vi "VSG_SET-GET_CW_1.00.vi"(4 "Set Delay after (ms)":i64 caption="Delay Time (s)", 5 "Skip(T)":bool, 6 "Freq Units":string(combo)="MHz", 7 "Timeout":u32=3000, 8 "error in":errorcluster {"code" format="%.0x"}, 9 "Set Freq (MHz) num":dbl, 10 "Set Freq (MHz)str":string, 11 "Session In":refnum<visa-resource-name>="TCPIP0::10.0.1.20::inst0::INSTR") -> (0 "error out":errorcluster {"code" format="%.0x"}, 1 "Get Freq (str)":string, 2 "Get Freq":dbl, 3 "Session Out":refnum<visa-resource-name>)   [LabVIEW 2018]
doc: "Sets the RF CF in MHz"
panel:
  in  "RO (T)":bool
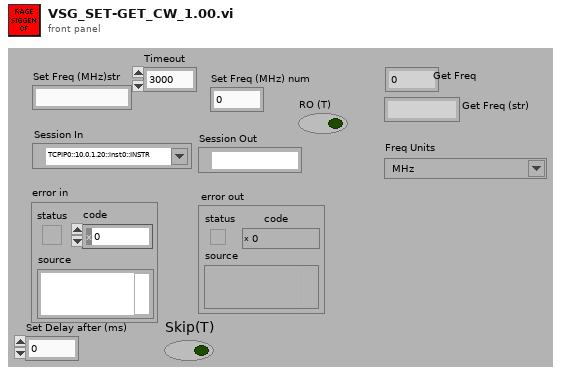
[diagram p1: front panel]
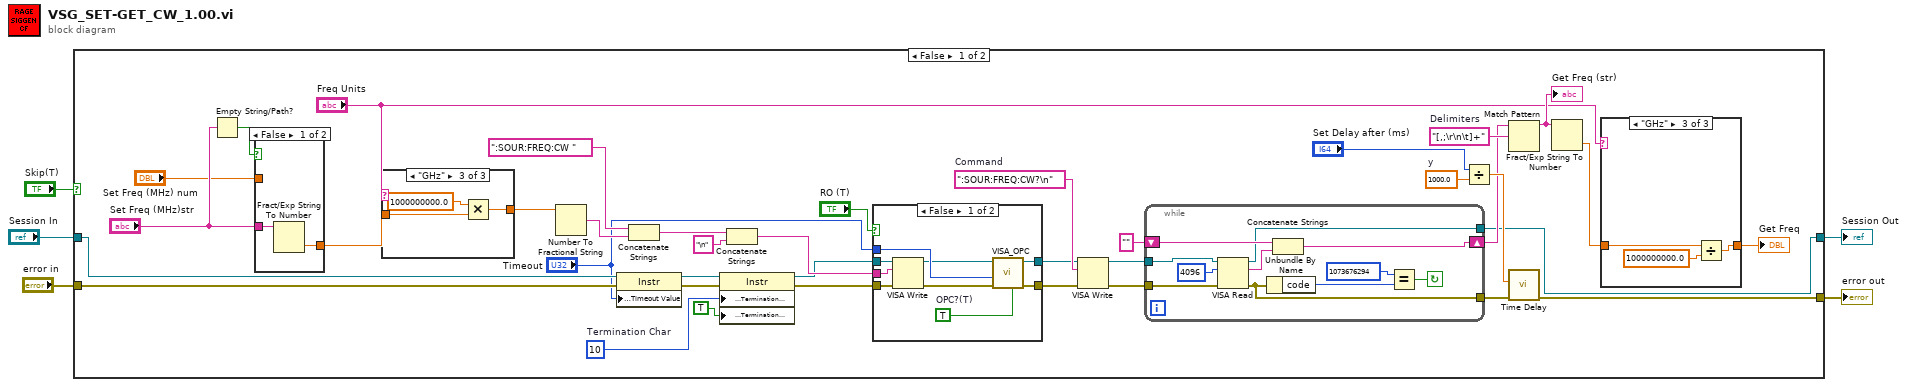
[diagram p0: block diagram]
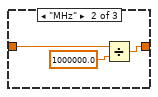
[diagram p4: hidden frame]
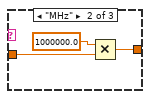
[diagram p6: hidden frame]
diagram:
  n1 = case shown="False" "Skip(T)" {
    tunnel: "error in" -> [w43 w83]
    tunnel: "Session In" -> [w42 w84]
    tunnel: [w6 w84] -> w3
    tunnel: [w16 w83] -> w2
    frame False {
      w13 = 1000.0  # y
      w33 = "[,;\r\n\t]+"  # Delimiters
      w34 = ":SOUR:FREQ:CW?\n"  # Command
      w39 = u8 10  # Termination Char
      n2 = Empty String/Path?(string/path="Set Freq (MHz)str") -> (empty?=w23:bool)
      n3 = case shown="False" w23 {
        tunnel: [w70 w71] -> w28
        tunnel: "Set Freq (MHz)str" -> [w69 _]
        tunnel: "Set Freq (MHz) num" -> [_ w71]
        frame False {
          n4 = Fract/Exp String To Number(string=w69) -> (number=w70:dbl)  [unwired: 3 in, 1 out]
        }
        frame True {
        }
      }
      n5 = case shown="\"GHz\"" "Freq Units" {
        tunnel: w28 -> [w62 w65 w68]
        tunnel: [w62 w63 w66] -> w26
        frame "Hz", Default {
        }
        frame "MHz" {
          n6 = Multiply(x=1000000.0, y=w65) -> (x*y=w63:dbl)
        }
        frame "GHz" {
          n7 = Multiply(x=1000000000.0, y=w68) -> (x*y=w66:dbl)
        }
      }
      n8 = Number To Fractional String(number=w26) -> (F-format string=w27:string)  [unwired: 3 in]
      n9 = property class="Instr"(reference=w42, error in=w43, "General Settings:Timeout Value"="Timeout") -> (reference out=w41:refnum<visa-resource-name>, error out=w40:errorcluster)
      n10 = Concatenate Strings(":SOUR:FREQ:CW " ("staticText"), w27) -> (w32:string)
      n11 = property class="Instr"(reference=w41, error in=w40, "Message Based Settings:Termination Character"=w39, "Message Based Settings:Termination Character Enable"=TRUE ("enable")) -> (reference out=w9:refnum<visa-resource-name>, error out=w11:errorcluster)
      n12 = Concatenate Strings(w32, "\n" ("StaticText")) -> (w30:string)
      n13 = case shown="False" "RO (T)" {
        tunnel: w11 -> [w52 w54]
        tunnel: w30 -> [w51 _]
        tunnel: w9 -> [w50 w53]
        tunnel: "Timeout" -> [w49 _]
        tunnel: [w48 w54] -> w12
        tunnel: [w44 w53] -> w8
        frame False {
          w45 = TRUE  # OPC?(T)
          n14 = VISA Write(VISA resource name=w50, write buffer=w51, error in (no error)=w52) -> (VISA resource name out=w47:refnum<visa-resource-name>, error out=w46:errorcluster)  [unwired: 1 out]
          n15 = call "VISA_OPC.vi"("OPC(T)"=w45, "error in"=w46, "Timeout"=w49, "Session In"=w47) -> ("error out"=w48:errorcluster, "Session Out"=w44:refnum<visa-resource-name>)  [unwired: 5 in, 1 out]
        }
        frame True {
        }
      }
      n16 = VISA Write(VISA resource name=w8, write buffer=w34, error in (no error)=w12) -> (VISA resource name out=w37:refnum<visa-resource-name>, error out=w36:errorcluster)  [unwired: 1 out]
      n17 = while {
        tunnel: w37 -> [w79]
        shift-right: [w73] -> w10
        shift-left: "" -> [w78]
        tunnel: w36 -> [w76]
        tunnel: [w75] -> w7
        tunnel: [w72] -> w6
        stop <- w74 continue-if-true
        n18 = VISA Read(VISA resource name=w79, byte count=u32 4096 ("byte count (0)"), error in (no error)=w76) -> (VISA resource name out=w72:refnum<visa-resource-name>, read buffer=w77:string, error out=w75:errorcluster)  [unwired: 1 out]
        n19 = Unbundle By Name(w75) -> ("code"=w81:i32)
        n20 = Concatenate Strings(w78, w77) -> (w73:string)
        n21 = Equal?(x=1073676294, y=w81) -> (x = y?=w74:bool)
      }
      n22 = Divide(x="Set Delay after (ms)", y=w13) -> (x/y=w14:dbl)
      n23 = Match Pattern(string=w10, regular expression=w33) -> (before substring=w20:string)  [unwired: 1 in, 3 out]
      "Get Freq (str)" <- w20
      n24 = call "Time Delay"("error in (no error)"=w7, "Delay Time (s)"=w14) -> ("error out"=w16:errorcluster)  [unwired: 9 in]
      n25 = Fract/Exp String To Number(string=w20) -> (number=w19:dbl)  [unwired: 3 in, 1 out]
      n26 = case shown="\"GHz\"" "Freq Units" {
        tunnel: [w55 w58 w61] -> w17
        tunnel: w19 -> [w55 w56 w59]
        frame "Hz", Default {
        }
        frame "MHz" {
          n27 = Divide(x=w56, y=1000000.0 ("x")) -> (x/y=w58:dbl)
        }
        frame "GHz" {
          n28 = Divide(x=w59, y=1000000000.0 ("x")) -> (x/y=w61:dbl)
        }
      }
      "Get Freq" <- w17
    }
    frame True {
    }
  }
  "error out" <- w2
  "Session Out" <- w3
